vi "Relay Command_TS.vi"(8 "error in (no error)":errorcluster, 11 "Relay Command":bool[](array[boolean])) -> (0 "error out":errorcluster, 3 "VISA Refnum out":refnum<visa-resource-name>)   [LabVIEW 2022 SP3]
uses:
  <vilib>/Instr/_visa.llb/VISA Flush IO Buffer Mask.ctl
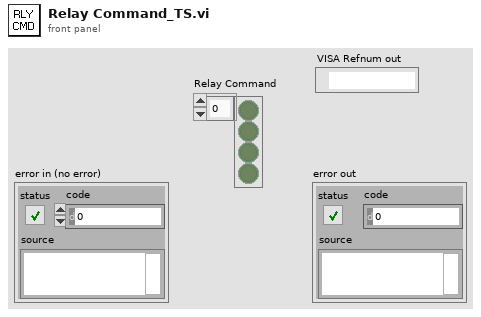
[diagram p1: front panel]
types:
  T1 = typedef "VISA Flush IO Buffer Mask.ctl" = u16
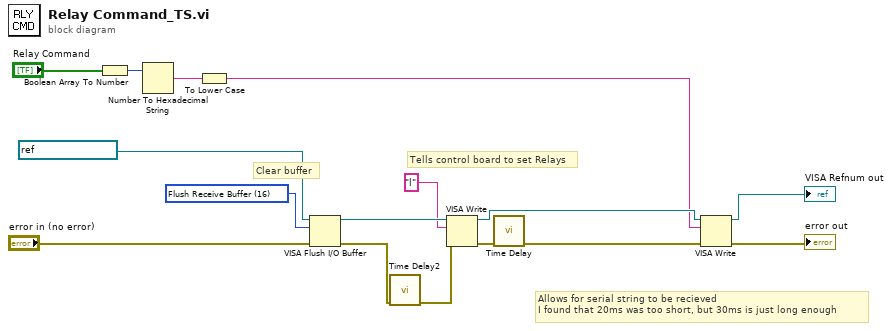
[diagram p0: block diagram]
diagram:
  w10 = T1 16 items=["Flush Receive Buffer"=16, "Write Transmit Buffer to Device"=32, "Flush Receive Buffer (No I/O)"=64, "Flush Transmit Buffer"=128] ("Mask")
  # "Clear buffer"
  # "Allows for serial string to be recieved\nI found that 20ms was too short, but 30ms is just long enough"
  # "Tells control board to set Relays"
  n1 = Boolean Array To Number(Boolean array="Relay Command") -> (number=w12:u32)
  n2 = Number To Hexadecimal String(2:w12) -> (0:w5:string)  [unwired: 1 in]
  n3 = To Lower Case(string=w5) -> (all lower case string=w4:string)
  n4 = VISA Flush I/O Buffer(VISA resource name=refnum<visa-resource-name> "ControlBoard", mask (16)=w10, error in (no error)="error in (no error)") -> (VISA resource name out=w15:refnum<visa-resource-name>, error out=w2:errorcluster)
  n5 = call "Time Delay2"("error in (no error)"=w2) -> ("error out"=w1:errorcluster)  [unwired: 10 in]
  n6 = VISA Write(VISA resource name=w15, write buffer="l", error in (no error)=w1) -> (VISA resource name out=w9:refnum<visa-resource-name>, error out=w14:errorcluster)  [unwired: 1 out]
  n7 = call "Time Delay"("error in (no error)"=w14) -> ("error out"=w8:errorcluster)  [unwired: 10 in]
  n8 = VISA Write(VISA resource name=w9, write buffer=w4, error in (no error)=w8) -> (VISA resource name out=→"VISA Refnum out":refnum<visa-resource-name>, error out=→"error out":errorcluster)  [unwired: 1 out]
